vi "Add_Next_Calib_Details.vi"(1 "% Change":dbl format="%.2f", 3 "Hours between calibrations":dbl format="%.2f", 4 "Instrument type":T1=enum."Cross wire velocity", 5 "Calib file Orig":path=path "/Hong(6%)/calib/XW Ch 1 7_10_02_5", 6 "Calib file New":path=path "/Hong(6%)/calib/XW Ch 1 7_10_02_6") -> (0 "Results Files Updated":bool)   [LabVIEW 2022 SP3]
uses:
  Controls/Cal_Inst_type.ctl
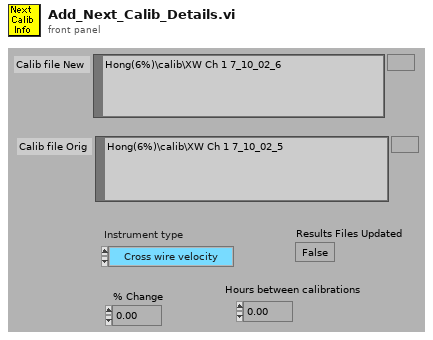
[diagram p1: front panel]
types:
  T1 = typedef "Cal_Inst_type.ctl" = enum16{"Propeller anemometer", "Pressure Transducer", "Hot wire", "Cross wire velocity", "Cross wire angle", "Generic Linear", "Generic Polynomial", "Poly Fit Special", "Fast FID", "Thermocouple", "Cold wire", "Pulsed Wire"}
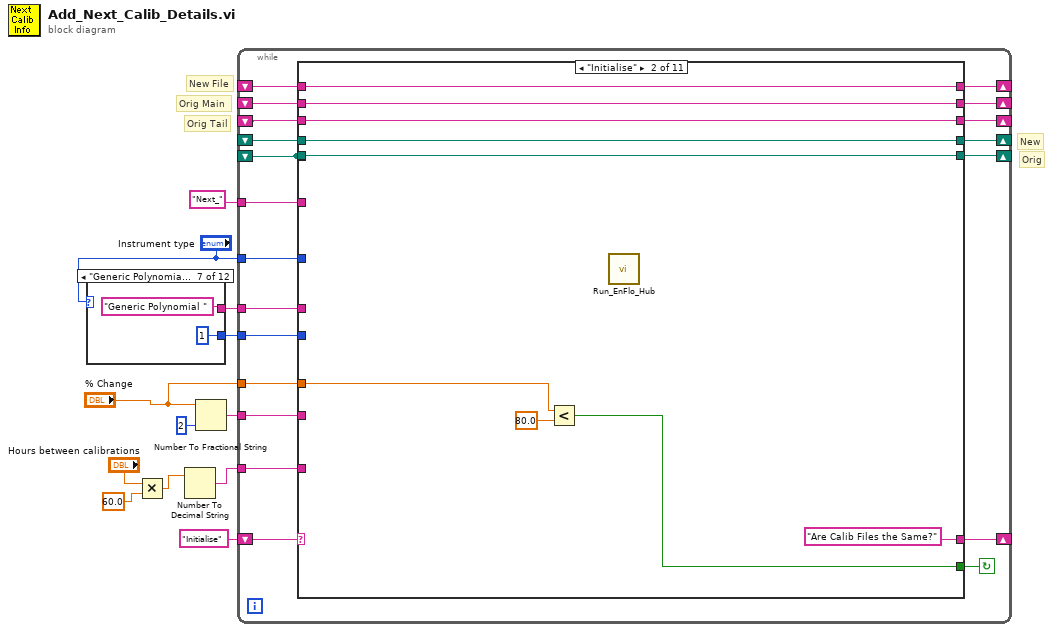
[diagram p0: block diagram]
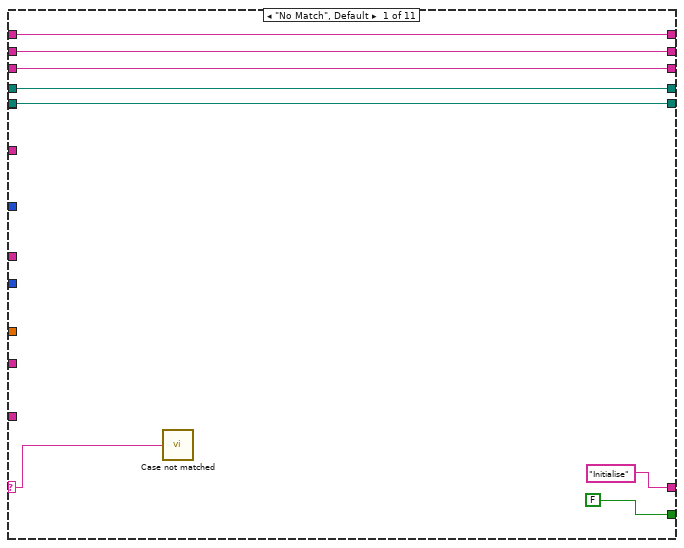
[diagram p2: hidden frame]
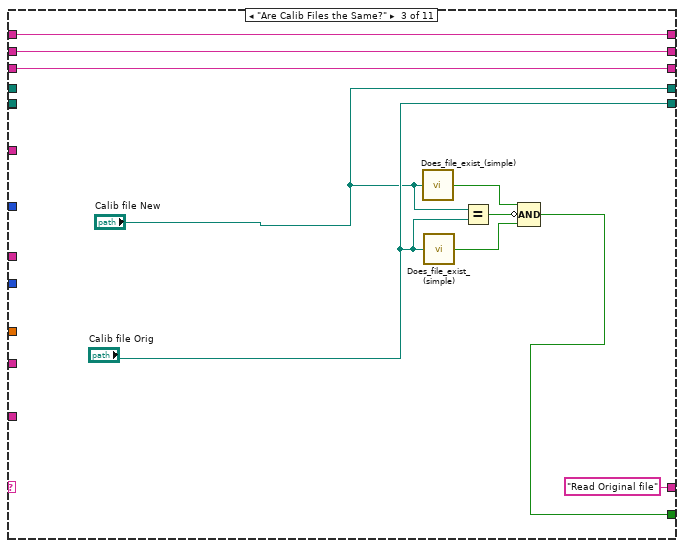
[diagram p3: hidden frame]
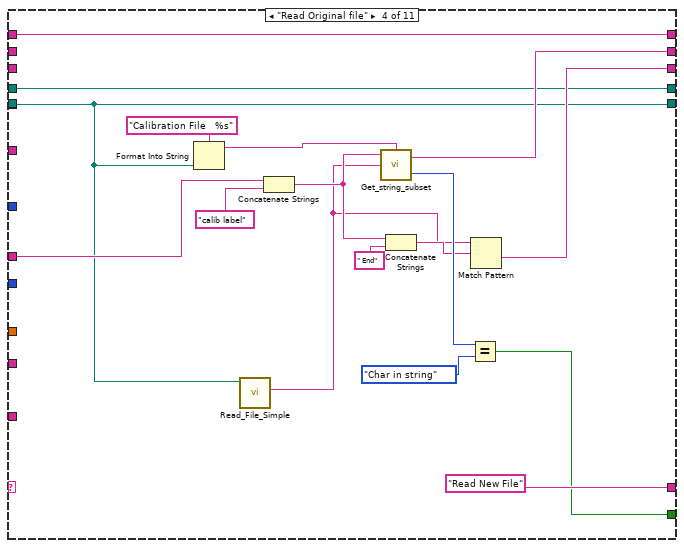
[diagram p4: hidden frame]
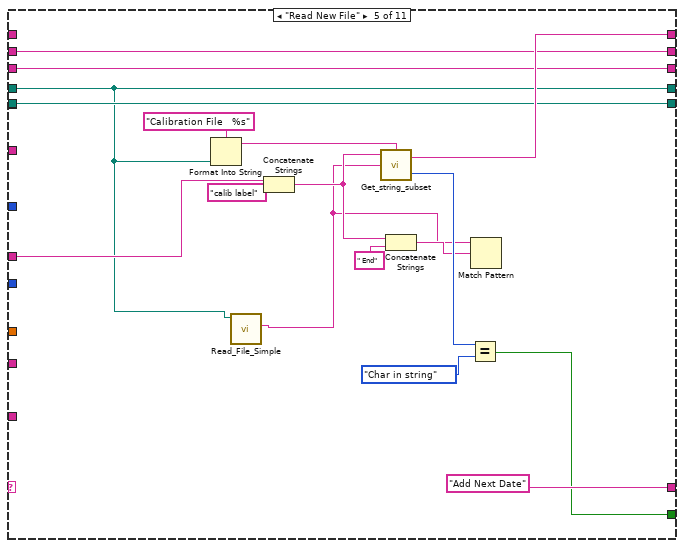
[diagram p5: hidden frame]
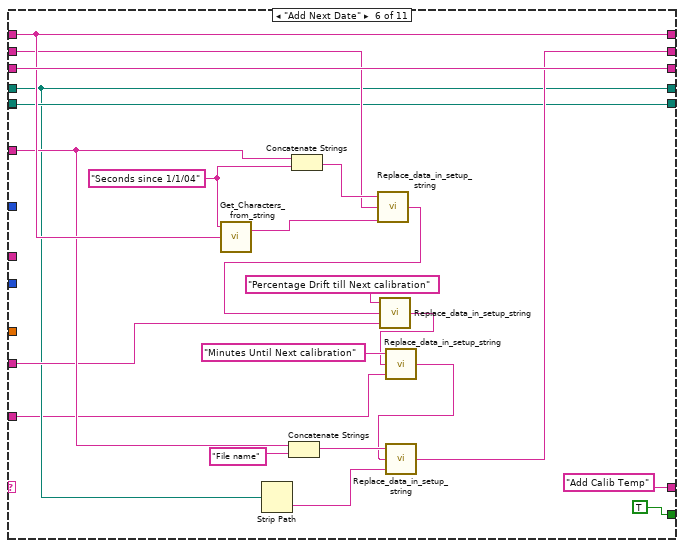
[diagram p6: hidden frame]
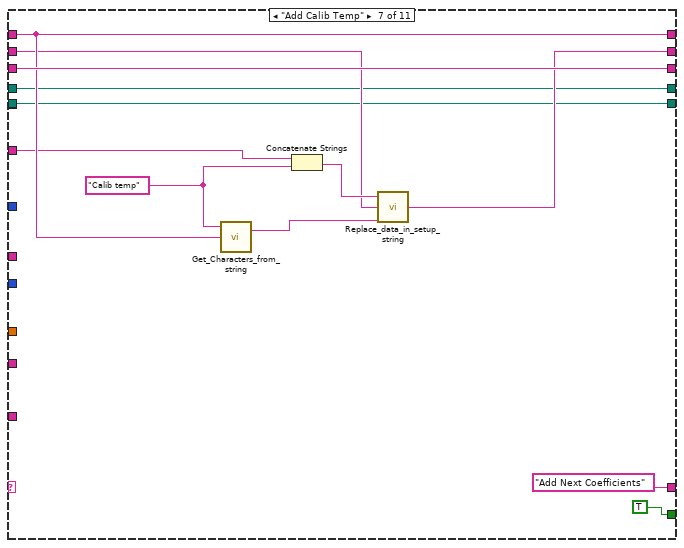
[diagram p7: hidden frame]
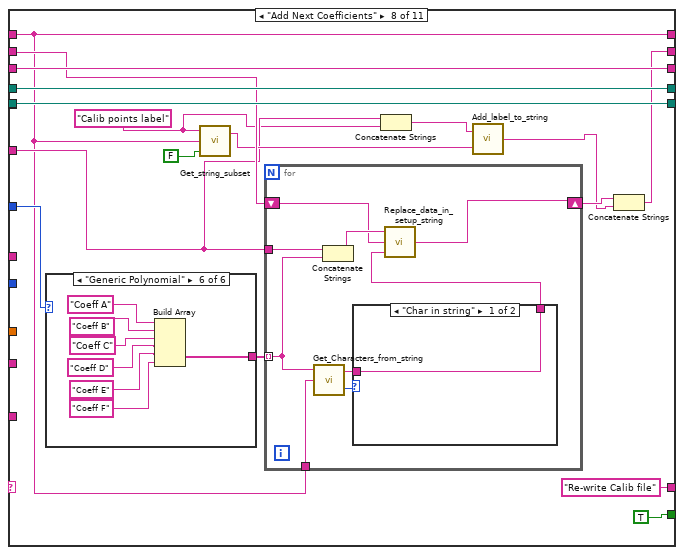
[diagram p8: hidden frame]
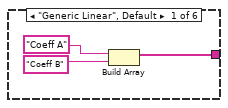
[diagram p9: hidden frame]
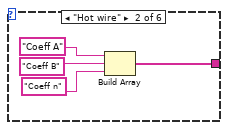
[diagram p10: hidden frame]
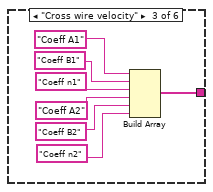
[diagram p11: hidden frame]
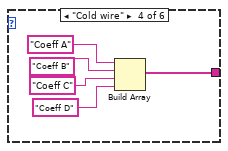
[diagram p12: hidden frame]
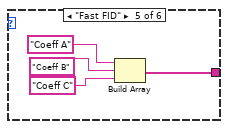
[diagram p13: hidden frame]
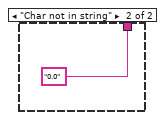
[diagram p14: hidden frame]
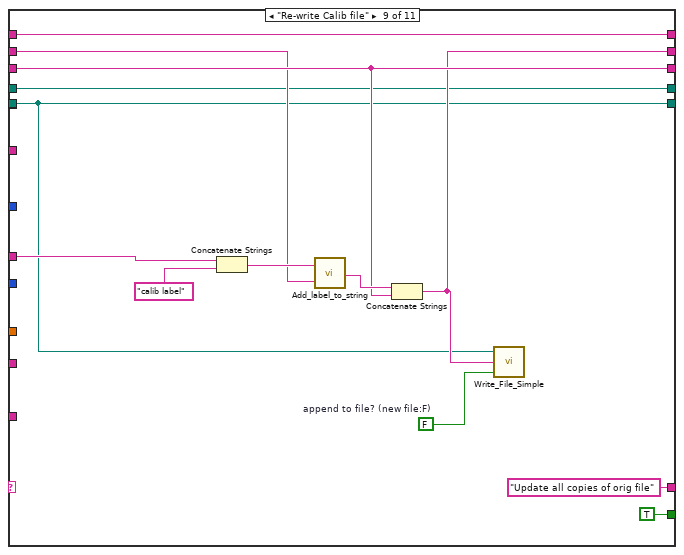
[diagram p15: hidden frame]
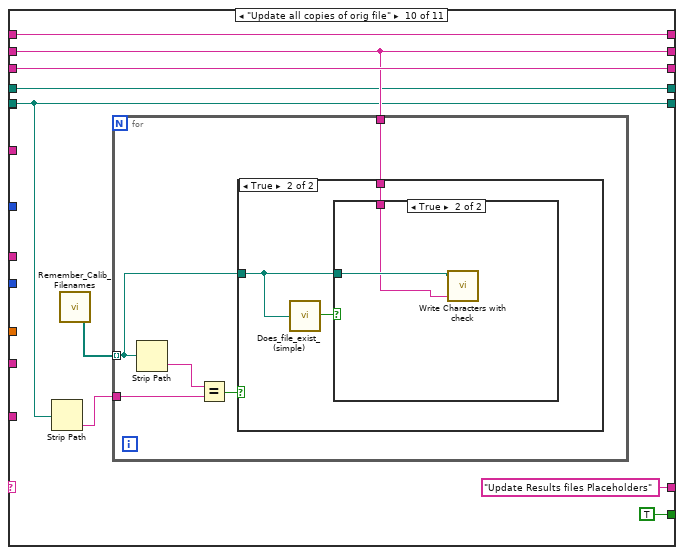
[diagram p16: hidden frame]
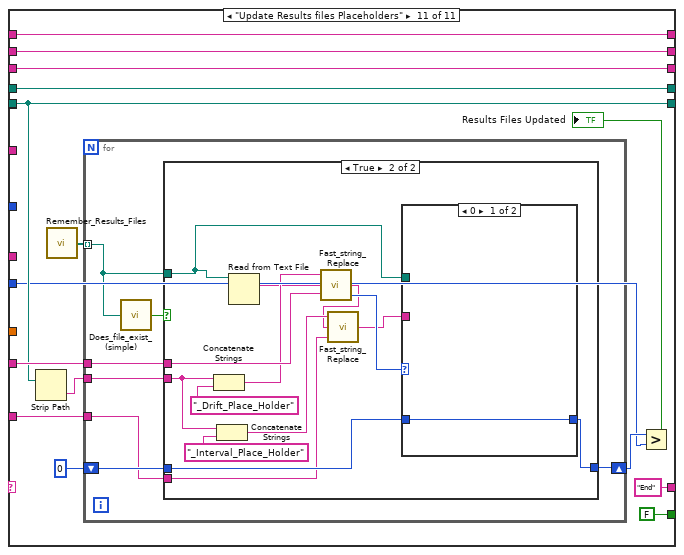
[diagram p19: hidden frame]
diagram:
  # "Orig"
  # "New"
  # "Orig Tail"
  # "New File"
  # "Orig Main"
  n1 = case shown="\"Generic Polynomial\"" "Instrument type" {
    tunnel: ["Prop " "Mano " "HW " "Cross wire velocity " "Cross wire angle " "Generic Inst " "Generic Polynomial " "Generic BackPoly " "Fast FID " "Thermocouple " "Cold wire " "Pulsed wire "] -> w10
    tunnel: [1 ("y") 1 ("y") 1 ("y") 1 ("y") 1 ("y") 1 ("y") 1 ("y") 1 ("y") 3 ("y") 1 ("y") 1 ("y") 1 ("y")] -> w2
    frame "Propeller anemometer" {
    }
    frame "Pressure Transducer" {
    }
    frame "Hot wire" {
    }
    frame "Cross wire velocity" {
    }
    frame "Cross wire angle" {
    }
    frame "Generic Linear" {
    }
    frame "Generic Polynomial" {
    }
    frame "Poly Fit Special" {
    }
    frame "Fast FID" {
    }
    frame "Thermocouple" {
    }
    frame "Cold wire" {
    }
    frame "Pulsed Wire" {
    }
  }
  n2 = Multiply(x="Hours between calibrations", y=60.0) -> (x*y=w4:dbl)
  n3 = Number To Decimal String(number=w4) -> (decimal integer string=w6:string)  [unwired: 1 out]
  n4 = Number To Fractional String(number="% Change", precision (6)=i16 2) -> (F-format string=w7:string)  [unwired: 2 out]
  n5 = while {
    shift-left: _ -> [w40]
    shift-right: [w42] -> _
    shift-left: _ -> [w43]
    shift-right: [w41] -> _
    tunnel: w7 -> [w44]
    tunnel: "Next_" -> [w45]
    tunnel: w10 -> [w46]
    shift-left: _ -> [w47]
    shift-right: [w48] -> _
    shift-left: _ -> [w49]
    shift-right: [w51] -> _
    tunnel: "Instrument type" -> [w53]
    shift-left: _ -> [w50]
    shift-right: [w52] -> _
    shift-left: "Initialise" -> [w54]
    shift-right: [w55] -> _
    tunnel: w6 -> [w39]
    tunnel: w2 -> [w38]
    tunnel: "% Change" -> [w37]
    stop <- w56 continue-if-true
    n6 = case shown="\"Initialise\"" w54 {
      selector: w54 -> [w57 _ _ _ _ _ _ _ _ _ _]
      tunnel: [FALSE w65 w76 w89 w106 TRUE TRUE TRUE TRUE TRUE FALSE] -> w56
      tunnel: ["Initialise" "Are Calib Files the Same?" "Read Original file" "Read New File" "Add Next Date" "Add Calib Temp" "Add Next Coefficients" "Re-write Calib file" "Update all copies of orig file" "Update Results files Placeholders" "End"] -> w55
      tunnel: w53 -> [_ _ _ _ _ _ _ w165 _ _ _]
      tunnel: [w62 w73 w83 w93 w115 w133 w145 w152 w220 w229 w254] -> w52
      tunnel: [w61 w71 w81 w91 w108 w134 w146 w168 w215 w228 w253] -> w51
      tunnel: w50 -> [w62 w73 w83 w93 _ w133 w145 w152 w220 w229 w254]
      tunnel: w49 -> [w61 w71 w81 _ w108 w134 w146 w168 w215 w228 w253]
      tunnel: [w60 w72 w82 w92 w109 w129 w142 w153 w212 w225 w251] -> w48
      tunnel: w47 -> [w60 w72 w82 _ w109 w132 w144 w161 w213 w225 w251]
      tunnel: w46 -> [_ _ _ w97 w112 _ _ _ w218 _ _]
      tunnel: w45 -> [_ _ _ _ _ w127 w143 w158 _ _ _]
      tunnel: w44 -> [_ _ _ _ _ w124 _ _ _ _ w249]
      tunnel: [w59 w69 "Calib file New" w88 w102 w122 w141 w163 w211 w224 w248] -> w41
      tunnel: [w58 w68 "Calib file Orig" w84 w105 w123 w140 w162 w210 w223 w247] -> w42
      tunnel: w40 -> [w58 w68 _ w84 w105 w123 w140 w162 w210 w223 _]
      tunnel: w43 -> [w59 w69 _ w88 w102 w122 w141 w163 w211 w224 w248]
      tunnel: w40 -> [_ _ _ _ _ _ _ _ _ _ w247]
      tunnel: w39 -> [_ _ _ _ _ w118 _ _ _ _ w245]
      tunnel: w38 -> [_ _ _ _ _ _ _ _ _ _ w242]
      tunnel: w37 -> [_ w67 _ _ _ _ _ _ _ _ _]
      frame "No Match", Default {
        n7 = call "Case not matched.vi"("Case Name not Matched"=w57) -> ()
      }
      frame "Initialise" {
        n8 = Less?(x=w67, y=80.0) -> (x < y?=w65:bool)
        n9 = call "Run_EnFlo_Hub.vi"() -> ()  [unwired: 1 in, 7 out]
      }
      frame "Are Calib Files the Same?" {
        n10 = call "Does_file_exist_(simple).vi"("Pathname"="Calib file New") -> ("exists?"=w78:bool)
        n11 = call "Does_file_exist_(simple).vi"("Pathname"="Calib file Orig") -> ("exists?"=w77:bool)
        n12 = Equal?(x="Calib file New", y="Calib file Orig") -> (x = y?=w79:bool)
        n13 = Compound Arithmetic op=AND(w78, invert w79, w77) -> (w76:bool)
      }
      frame "Read Original file" {
        n14 = Format Into String(format string="Calibration File   %s", w84) -> (resulting string=w85:string)  [unwired: 2 in, 1 out]
        n15 = call "Read_File_Simple.vi"("Filename"=w84) -> ("string"=w87:string)  [unwired: 2 in, 7 out]
        n16 = Concatenate Strings(w97, "calib label") -> (w94:string)
        n17 = call "Get_string_subset.vi"("String Name"=w85, "String to split"=w87, "File Label"=w94) -> ("Status"=w98:enum16{"Char in string", "Char not in string"}, "Output string"=w92:string)  [unwired: 1 in]
        n18 = Concatenate Strings(w94, " End") -> (w95:string)
        n19 = Equal?(x=w98, y=enum16{"Char in string", "Char not in string"}."Char in string" ("Status")) -> (x = y?=w89:bool)
        n20 = Match Pattern(string=w87, regular expression=w95) -> (after substring=w91:string)  [unwired: 4 out]
      }
      frame "Read New File" {
        n21 = Format Into String(format string="Calibration File   %s", w102) -> (resulting string=w101:string)  [unwired: 2 in, 1 out]
        n22 = call "Read_File_Simple.vi"("Filename"=w102) -> ("string"=w104:string)  [unwired: 2 in, 7 out]
        n23 = Concatenate Strings(w112, "calib label") -> (w107:string)
        n24 = call "Get_string_subset.vi"("String Name"=w101, "String to split"=w104, "File Label"=w107) -> ("Status"=w114:enum16{"Char in string", "Char not in string"}, "Output string"=w115:string)  [unwired: 1 in]
        n25 = Concatenate Strings(w107, " End") -> (w110:string)
        n26 = Equal?(x=w114, y=enum16{"Char in string", "Char not in string"}."Char in string" ("Status")) -> (x = y?=w106:bool)
        n27 = Match Pattern(string=w104, regular expression=w110) -> ()  [unwired: 5 out]
      }
      frame "Add Next Date" {
        w137 = "Seconds since 1/1/04"
        n28 = call "Get_Characters_from_string.vi"("Input string"=w133, "Variable name"=w137) -> ("Value"=w135:string)  [unwired: 1 in, 1 out]
        n29 = Strip Path(path=w122) -> (name=w125:string)  [unwired: 1 out]
        n30 = Concatenate Strings(w127, "File name" ("Variable name")) -> (w126:string)
        n31 = Concatenate Strings(w127, w137) -> (w136:string)
        n32 = call "Replace_data_in_setup_string.vi"("New data string"=w135, "Input string"=w132, "Variable name"=w136) -> ("Appended string"=w130:string)
        n33 = call "Replace_data_in_setup_string.vi"("New data string"=w124, "Input string"=w130, "Variable name"="Percentage Drift till Next calibration") -> ("Appended string"=w120:string)
        n34 = call "Replace_data_in_setup_string.vi"("New data string"=w118, "Input string"=w120, "Variable name"="Minutes Until Next calibration") -> ("Appended string"=w119:string)
        n35 = call "Replace_data_in_setup_string.vi"("New data string"=w125, "Input string"=w119, "Variable name"=w126) -> ("Appended string"=w129:string)
      }
      frame "Add Calib Temp" {
        w149 = "Calib temp"
        n36 = call "Get_Characters_from_string.vi"("Input string"=w145, "Variable name"=w149) -> ("Value"=w147:string)  [unwired: 1 in, 1 out]
        n37 = Concatenate Strings(w143, w149) -> (w148:string)
        n38 = call "Replace_data_in_setup_string.vi"("New data string"=w147, "Input string"=w144, "Variable name"=w148) -> ("Appended string"=w142:string)
      }
      frame "Add Next Coefficients" {
        w157 = "Calib points label"
        n39 = case shown="\"Generic Polynomial\"" w165 {
          tunnel: [w169 w172 w176 w183 w188 w195] -> w164
          frame "Generic Linear", Default {
            n40 = Build Array("Coeff A", "Coeff B") -> (w169:string[])
          }
          frame "Hot wire" {
            n41 = Build Array("Coeff A", "Coeff B", "Coeff n") -> (w172:string[])
          }
          frame "Cross wire velocity" {
            n42 = Build Array("Coeff A1", "Coeff B1", "Coeff n1", "Coeff A2", "Coeff B2", "Coeff n2") -> (w176:string[])
          }
          frame "Cold wire" {
            n43 = Build Array("Coeff A", "Coeff B", "Coeff C", "Coeff D") -> (w183:string[])
          }
          frame "Fast FID" {
            n44 = Build Array("Coeff A", "Coeff B", "Coeff C") -> (w188:string[])
          }
          frame "Generic Polynomial" {
            n45 = Build Array("Coeff A", "Coeff B", "Coeff C", "Coeff D", "Coeff E", "Coeff F") -> (w195:string[])
          }
        }
        n46 = call "Get_string_subset.vi"("Show Dialog?"=FALSE, "String to split"=w152, "File Label"=w157) -> ("Output string"=w159:string)  [unwired: 1 in, 1 out]
        n47 = for {
          tunnel: w164 -> [w206] mode=indexing
          tunnel: w158 -> [w207]
          shift-right: [w203] -> w155
          shift-left: w161 -> [w204]
          tunnel: w152 -> [w199]
          n48 = call "Get_Characters_from_string.vi"("Input string"=w199, "Variable name"=w206) -> ("Status"=w202:enum16{"Char in string", "Char not in string"}, "Value"=w201:string)  [unwired: 1 in]
          n49 = Concatenate Strings(w207, w206) -> (w205:string)
          n50 = case shown="\"Char in string\"" w202 {
            tunnel: w201 -> [w208 _]
            tunnel: [w208 "0.0"] -> w200
            frame "Char in string" {
            }
            frame "Char not in string" {
            }
          }
          n51 = call "Replace_data_in_setup_string.vi"("New data string"=w200, "Input string"=w204, "Variable name"=w205) -> ("Appended string"=w203:string)
        }
        n52 = Concatenate Strings(w158, w157) -> (w156:string)
        n53 = call "Add_label_to_string.vi"("String to write"=w159, "File Label"=w156) -> ("Output string"=w154:string)
        n54 = Concatenate Strings(w155, w154) -> (w153:string)
      }
      frame "Re-write Calib file" {
        w214 = FALSE  # append to file? (new file:F)
        n55 = Concatenate Strings(w218, "calib label") -> (w217:string)
        n56 = call "Add_label_to_string.vi"("String to write"=w213, "File Label"=w217) -> ("Output string"=w216:string)
        n57 = Concatenate Strings(w216, w215) -> (w212:string)
        n58 = call "Write_File_Simple.vi"("append to file? (new file:F)"=w214, "character string"=w212, "file path"=w210) -> ()  [unwired: 2 out]
      }
      frame "Update all copies of orig file" {
        n59 = Strip Path(path=w223) -> (name=w226:string)  [unwired: 1 out]
        n60 = call "Remember_Calib_Filenames.vi"() -> ("List of Filenames"=w227:path[])  [unwired: 1 in]
        n61 = for {
          tunnel: w227 -> [w233] mode=indexing
          tunnel: w226 -> [w235]
          tunnel: w225 -> [w232]
          n62 = Strip Path(path=w233) -> (name=w236:string)  [unwired: 1 out]
          n63 = Equal?(x=w236, y=w235) -> (x = y?=w234:bool)
          n64 = case shown="True" w234 {
            tunnel: w233 -> [_ w238]
            tunnel: w232 -> [_ w239]
            frame False {
            }
            frame True {
              n65 = call "Does_file_exist_(simple).vi"("Pathname"=w238) -> ("exists?"=w237:bool)
              n66 = case shown="True" w237 {
                tunnel: w238 -> [_ w241]
                tunnel: w239 -> [_ w240]
                frame False {
                }
                frame True {
                  n67 = call "Write Characters with check.vi"("String to Write"=w240, "file (use dialog)"=w241) -> ()  [unwired: 2 in, 1 out]
                }
              }
            }
          }
        }
      }
      frame "Update Results files Placeholders" {
        n68 = Strip Path(path=w247) -> (name=w250:string)  [unwired: 1 out]
        n69 = call "Remember_Results_Files.vi"() -> ("List of Filenames"=w252:path[])  [unwired: 1 in]
        n70 = for {
          tunnel: w252 -> [w261] mode=indexing
          tunnel: w250 -> [w263]
          tunnel: w249 -> [w262]
          shift-right: [w257] -> w244
          shift-left: 0 -> [w259]
          tunnel: w245 -> [w258]
          n71 = call "Does_file_exist_(simple).vi"("Pathname"=w261) -> ("exists?"=w260:bool)
          n72 = case shown="True" w260 {
            tunnel: w263 -> [_ w271]
            tunnel: w262 -> [_ w278]
            tunnel: w261 -> [_ w266]
            tunnel: [w264 w274] -> w257
            tunnel: w259 -> [w264 w273]
            tunnel: w258 -> [_ w267]
            frame False {
            }
            frame True {
              n73 = Concatenate Strings(w271, "_Drift_Place_Holder" ("Substring")) -> (w276:string)
              n74 = Concatenate Strings(w271, "_Interval_Place_Holder" ("Substring")) -> (w270:string)
              n75 = Read from Text File(file (use dialog)=w266) -> (text=w265:string)  [unwired: 3 in, 3 out]
              n76 = call "Fast_string_Replace.vi"("Replace match with:"=w278, "Input String"=w265, "matchThis"=w276) -> ("Number Found"=w275:i32, "Output String"=w269:string)  [unwired: 1 in]
              n77 = call "Fast_string_Replace.vi"("Replace match with:"=w267, "Input String"=w269, "matchThis"=w270) -> ("Output String"=w268:string)  [unwired: 1 in, 1 out]
              n78 = case shown="0" w275 {
                tunnel: w266 -> [_ w281]
                tunnel: w268 -> [_ w280]
                tunnel: [w279 w282] -> w274
                tunnel: w273 -> [w279 w283]
                frame 0 {
                }
                frame 1, Default {
                  n79 = Increment(x=w283) -> (x+1=w282:i32)
                  n80 = call "Write Characters with check.vi"("String to Write"=w280, "file (use dialog)"=w281) -> ()  [unwired: 2 in, 1 out]
                }
              }
            }
          }
        }
        n81 = Greater?(x=w244, y=w242) -> (0:→"Results Files Updated":bool)
      }
    }
  }
